vi "raise Height recieve.vi"(8 "error in (no error)":errorcluster, 10 "stop?":bool) -> (0 "error out":errorcluster, 2 "Height_cm":dbl)   [LabVIEW 2019]
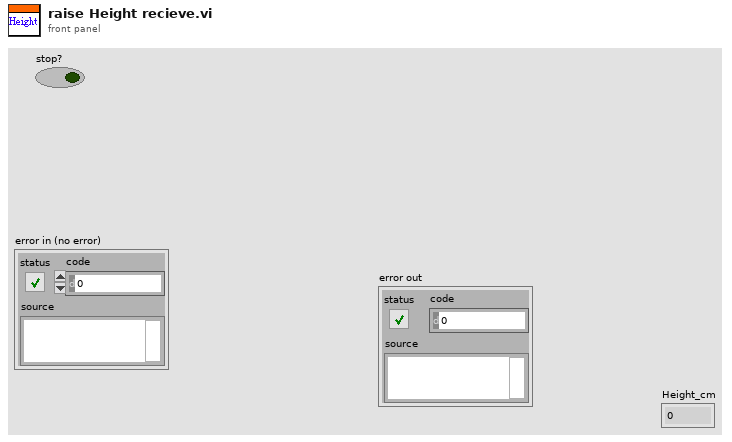
[diagram p1: front panel]
types:
  T1 = cluster{"read mode":enum16{"polling", "blocking"}, "write mode":enum16{"polling", "blocking"}}
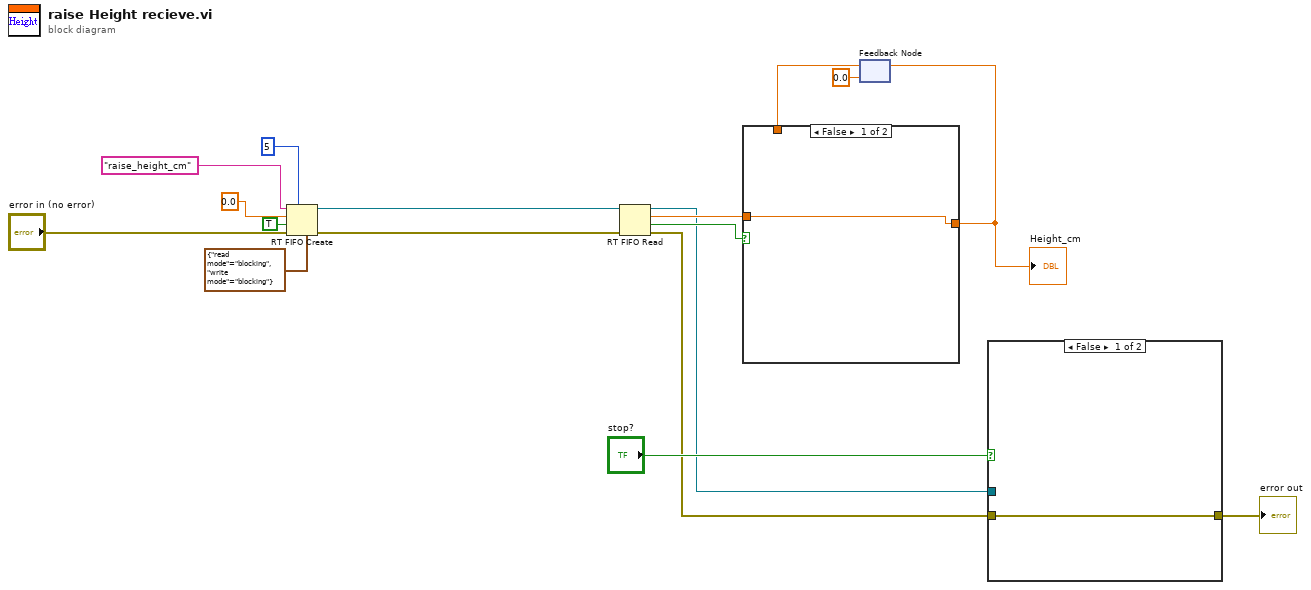
[diagram p0: block diagram]
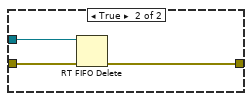
[diagram p2: hidden frame]
diagram:
  n1 = RT FIFO Create(0:"raise_height_cm" ("name (unnamed)"), 1:0.0, 2:TRUE ("create if not found? (T)"), 3:"error in (no error)", 4:u32 5 ("size (10)"), 7:T1 {"read mode"=enum."blocking", "write mode"=enum."blocking"} ("r/w modes (polling,polling)")) -> (8:w10:refnum<k33>, 11:w9:errorcluster)  [unwired: 2 in, 1 out]
  n2 = RT FIFO Read(0:w10, 3:w9) -> (8:w2:refnum<k33>, 9:w5:dbl, 10:w8:bool, 11:w3:errorcluster)  [unwired: 2 in, 1 out]
  n3 = feedback #1(0.0) -> (w6:dbl)
  n4 = case shown="False" w8 {
    tunnel: [w18 w19] -> w7
    tunnel: w6 -> [_ w19]
    tunnel: w5 -> [w18 _]
    frame False {
    }
    frame True {
    }
  }
  "Height_cm" <- w7
  n5 = feedback-in #1(w7) -> ()
  n6 = case shown="False" "stop?" {
    tunnel: w3 -> [w20 w23]
    tunnel: w2 -> [_ w22]
    tunnel: [w20 w21] -> w1
    frame False {
    }
    frame True {
      n7 = RT FIFO Delete(0:w22, 3:w23) -> (11:w21:errorcluster)  [unwired: 1 in]
    }
  }
  "error out" <- w1
